vi "Flatten I16.vi"(3 "I16":i16, 4 "Endian":T1) -> (5 "Flat Data":u8[](array[numeric]) format="%.0x")   [LabVIEW 2021, in "DataTypes_CIF_U.lvlib"]
uses:
  Endian.ctl
  DataTypes_CIF_U.lvlib
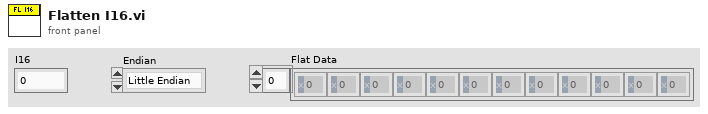
[diagram p1: front panel]
types:
  T1 = typedef "DataTypes_CIF_U.lvlib/Endian.ctl" = enum16{"Little Endian", "Big Endian"}
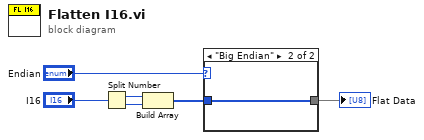
[diagram p0: block diagram]
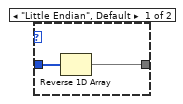
[diagram p2: hidden frame]
diagram:
  n1 = Split Number(x="I16") -> (hi(x)=w5:u8, lo(x)=w6:u8)
  n2 = Build Array(w5, w6) -> (w4:u8[])
  n3 = case shown="\"Big Endian\"" "Endian" {
    tunnel: w4 -> [w8 w9]
    tunnel: [w7 w9] -> w2
    frame "Little Endian", Default {
      n4 = Reverse 1D Array(array=w8) -> (reversed array=w7:u8[])
    }
    frame "Big Endian" {
    }
  }
  "Flat Data" <- w2
